vi "ReadInlineCNode.vi"(1 "reference":refnum<vi>) -> (0 "InlineCNode":T5)   [LabVIEW 2013]
uses:
  <vilib>/Utility/miscctls.llb/LVBoundsTypeDef.ctl
  <vilib>/Utility/miscctls.llb/LVPositionTypeDef.ctl
  <vilib>/Utility/miscctls.llb/LVRectTypeDef.ctl
  <vilib>/Utility/miscctls.llb/LVBreakpointStatusEnum.ctl
panel:
  out "error out 21":errorcluster
  out "error out 20":errorcluster
  out "error out 19":errorcluster
  out "error out 18":errorcluster
  out "error out 17":errorcluster
  out "error out 16":errorcluster
  out "error out 15":errorcluster
  out "error out 14":errorcluster
  out "error out 13":errorcluster
  out "error out 12":errorcluster
  out "error out 11":errorcluster
  out "error out 10":errorcluster
  out "error out 9":errorcluster
  out "error out 8":errorcluster
  out "error out 7":errorcluster
  out "error out 6":errorcluster
  out "error out 5":errorcluster
  out "error out 4":errorcluster
  out "error out 3":errorcluster
  out "error out 2":errorcluster
  out "error out":errorcluster
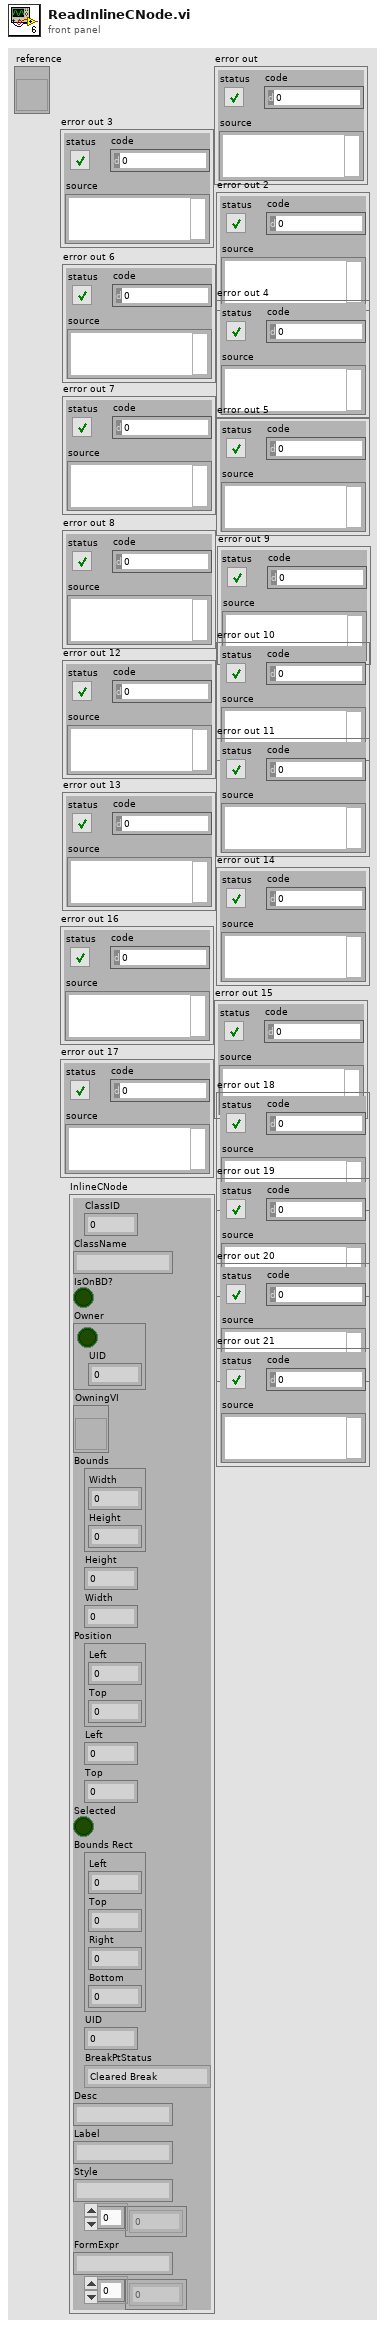
[diagram p1: front panel]
types:
  T1 = typedef "LVBoundsTypeDef.ctl" = cluster{"Width":u32, "Height":u32}
  T2 = typedef "LVPositionTypeDef.ctl" = cluster{"Left":i32, "Top":i32}
  T3 = typedef "LVRectTypeDef.ctl" = cluster{"Left":i16, "Top":i16, "Right":i16, "Bottom":i16}
  T4 = typedef "LVBreakpointStatusEnum.ctl" = enum8{"Cleared Break", "Enabled Break", "Disabled Break"}
  T5 = cluster{"ClassID":u32, "ClassName":string, "IsOnBD?":bool, "Owner":cluster{bool, "UID":i32}, "OwningVI":refnum<vi>, "Bounds":T1, "Height":u32, "Width":u32, "Position":T2, "Left":i32, "Top":i32, "Selected":bool, "Bounds Rect":T3, "UID":i32, "BreakPtStatus":T4, "Desc":string, "Label":string, "Style":string, "Terms[]":i32[], "FormExpr":string, "FormulaParameters[]":i32[]}
  T6 = cluster{"ClassID":u32, "ClassName":string, "IsOnBD?":bool, "Cluster":cluster{bool, "UID":i32}, "OwningVI":refnum<vi>, "Bounds":T1, "Height":u32, "Width":u32, "Position":T2, "Left":i32, "Top":i32, "Selected":bool, "Bounds Rect":T3, "UID":i32, "BreakPtStatus":T4, "Desc":string, "Text":string, "Style":string, i32[], "FormExpr":string, i32[]}
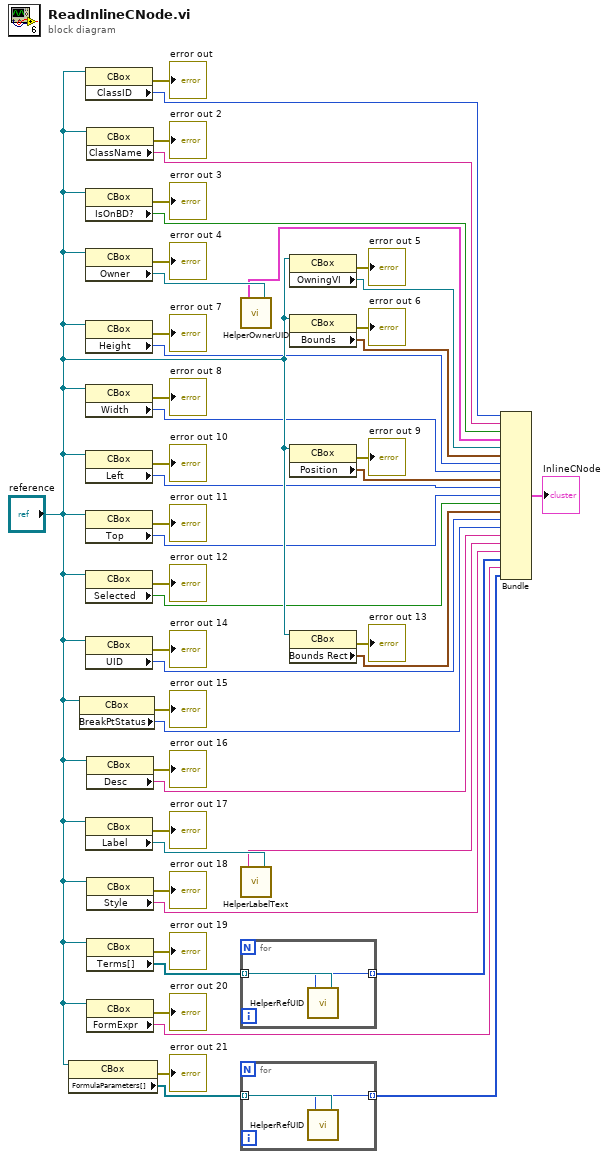
[diagram p0: block diagram]
diagram:
  n1 = property class="CBox"(reference="reference") -> (error out=→"error out 21":errorcluster, "FormulaParameters[]"=w3:refnum<vi>[])  [unwired: 1 in, 1 out]
  n2 = property class="CBox"(reference="reference") -> (error out=→"error out 15":errorcluster, "BreakPtStatus"=w17:T4)  [unwired: 1 in, 1 out]
  n3 = property class="CBox"(reference="reference") -> (error out=→"error out":errorcluster, "ClassID"=w46:u32)  [unwired: 1 in, 1 out]
  n4 = property class="CBox"(reference="reference") -> (error out=→"error out 3":errorcluster, "IsOnBD?"=w42:bool)  [unwired: 1 in, 1 out]
  n5 = property class="CBox"(reference="reference") -> (error out=→"error out 4":errorcluster, "Owner"=w40:refnum<vi>)  [unwired: 1 in, 1 out]
  n6 = property class="CBox"(reference="reference") -> (error out=→"error out 7":errorcluster, "Height"=w33:u32)  [unwired: 1 in, 1 out]
  n7 = property class="CBox"(reference="reference") -> (error out=→"error out 8":errorcluster, "Width"=w31:u32)  [unwired: 1 in, 1 out]
  n8 = property class="CBox"(reference="reference") -> (error out=→"error out 10":errorcluster, "Left"=w27:i32)  [unwired: 1 in, 1 out]
  n9 = property class="CBox"(reference="reference") -> (error out=→"error out 11":errorcluster, "Top"=w25:i32)  [unwired: 1 in, 1 out]
  n10 = property class="CBox"(reference="reference") -> (error out=→"error out 12":errorcluster, "Selected"=w23:bool)  [unwired: 1 in, 1 out]
  n11 = property class="CBox"(reference="reference") -> (error out=→"error out 14":errorcluster, "UID"=w19:i32)  [unwired: 1 in, 1 out]
  n12 = property class="CBox"(reference="reference") -> (error out=→"error out 17":errorcluster, "Label"=w13:refnum<vi>)  [unwired: 1 in, 1 out]
  n13 = property class="CBox"(reference="reference") -> (error out=→"error out 2":errorcluster, "ClassName"=w44:string)  [unwired: 1 in, 1 out]
  n14 = property class="CBox"(reference="reference") -> (error out=→"error out 16":errorcluster, "Desc"=w15:string)  [unwired: 1 in, 1 out]
  n15 = property class="CBox"(reference="reference") -> (error out=→"error out 18":errorcluster, "Style"=w10:string)  [unwired: 1 in, 1 out]
  n16 = property class="CBox"(reference="reference") -> (error out=→"error out 19":errorcluster, "Terms[]"=w8:refnum<vi>[])  [unwired: 1 in, 1 out]
  n17 = property class="CBox"(reference="reference") -> (error out=→"error out 20":errorcluster, "FormExpr"=w5:string)  [unwired: 1 in, 1 out]
  n18 = call "HelperOwnerUID.vi"("Generic in"=w40) -> ("Cluster"=w39:cluster{bool, "UID":i32})
  n19 = call "HelperLabelText.vi"("Text in"=w13) -> ("Text"=w12:string)
  n20 = for {
    tunnel: w8 -> [w50] mode=indexing
    tunnel: [w49] -> w7 mode=indexing
    n21 = call "HelperRefUID.vi"("Text in"=w50) -> ("UID"=w49:i32)
  }
  n22 = for {
    tunnel: w3 -> [w52] mode=indexing
    tunnel: [w51] -> w2 mode=indexing
    n23 = call "HelperRefUID.vi"("Text in"=w52) -> ("UID"=w51:i32)
  }
  n24 = property class="CBox"(reference="reference") -> (error out=→"error out 5":errorcluster, "OwningVI"=w37:refnum<vi>)  [unwired: 1 in, 1 out]
  n25 = property class="CBox"(reference="reference") -> (error out=→"error out 6":errorcluster, "Bounds"=w35:T1)  [unwired: 1 in, 1 out]
  n26 = property class="CBox"(reference="reference") -> (error out=→"error out 9":errorcluster, "Position"=w29:T2)  [unwired: 1 in, 1 out]
  n27 = property class="CBox"(reference="reference") -> (error out=→"error out 13":errorcluster, "Bounds Rect"=w21:T3)  [unwired: 1 in, 1 out]
  n28 = Bundle("ClassID"=w46, "ClassName"=w44, "IsOnBD?"=w42, "Cluster"=w39, "OwningVI"=w37, "Bounds"=w35, "Height"=w33, "Width"=w31, "Position"=w29, "Left"=w27, "Top"=w25, "Selected"=w23, "Bounds Rect"=w21, "UID"=w19, "BreakPtStatus"=w17, "Desc"=w15, "Text"=w12, "Style"=w10, w7, "FormExpr"=w5, w2) -> (→"InlineCNode":T6)  [unwired: 1 in]
